vi "XIPIN_LTE_Fast_Fourier_Transform_1_0.vi"   [LabVIEW 2017]
doc: "The LTE Fast Fourier Transform LogiCORE(TM) implements all transform lengths required by the 3GPP LTE specification, including the 1536-point transform for 15 MHz bandwidths. The transform length, transform direction, cyclic prefix length and scaling schedule may be configured on a per-frame basis.\n------------------------------------\n<b>Need License</b> : Yes"
uses:
  <vilib>/rvi/XilinxIP/XIPIN_XNode/niFpgaXIPIN.xnode
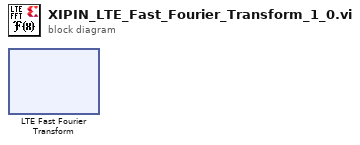
[diagram p0: block diagram]
diagram:
  n1 = xnode ("LTE Fast Fourier Transform")() -> ()
